vi "ldr motor sir.vi"() -> ()   [LabVIEW 2020]
uses:
  <vilib>/MakerHub/LINX/Private/Device/Type Defs/Stimulus Pulse.ctl
  <vilib>/MakerHub/LINX/Public/Peripherals/Analog/Analog Read 1 Chan.vi
  <vilib>/MakerHub/LINX/Public/Peripherals/Digital/Digital Write 1 Chan.vi
  <vilib>/MakerHub/LINX/Public/Peripherals/PWM/PWM Set Duty Cycle 1 Chan.vi
  <vilib>/MakerHub/LINX/Public/Peripherals/Analog/Analog Read N Chans.vi
  <vilib>/MakerHub/LINX/Public/Peripherals/Digital/Digital Write N Chans.vi
  <vilib>/MakerHub/LINX/Private/Local IO/LinxAnalogRead.vi
  <vilib>/MakerHub/LINX/Public/Utilities/Check Channel.vi
  <vilib>/MakerHub/LINX/Private/Local IO/LinxDigitalWrite.vi
  <vilib>/MakerHub/LINX/Public/Utilities/Open Serial.vi
  <vilib>/MakerHub/LINX/Private/Utilties/Generate Error.vi
  <vilib>/MakerHub/LINX/Public/Peripherals/PWM/PWM Set Duty Cycle N Chans.vi
  <vilib>/MakerHub/LINX/Private/Device/Device.lvlib
  <vilib>/MakerHub/LINX/LMH-LINX.lvlib
panel:
  in  "Serial Port":refnum<visa-resource-name>="N/A"
  in  "stop of ldr while":bool
  out "Light Intensity":dbl
  out "voltage across ldr":dbl
  in  "Knob":dbl(knob) scale=0.0..1.0
  out "Pulse Width (uS)":u32
  out "U1 Distance(cm)":u32
  out "Waveform Chart u1":dbl(graph)
  in  "Trigger":u8
  in  "Echo":u8
  in  "LDR Analog pin":u8
  in  "IN2 Motor":u8
  in  "Enable PWM Channel for  motor":u8
  in  "Trigger 2":u8
  in  "Echo 2":u8
  out "Pulse Width (uS) 2":u32
  out "U1 Distance(cm) 2":u32
  out "Waveform Chart u1\n 2":dbl(graph)
  in  "IN1 Motor":u8
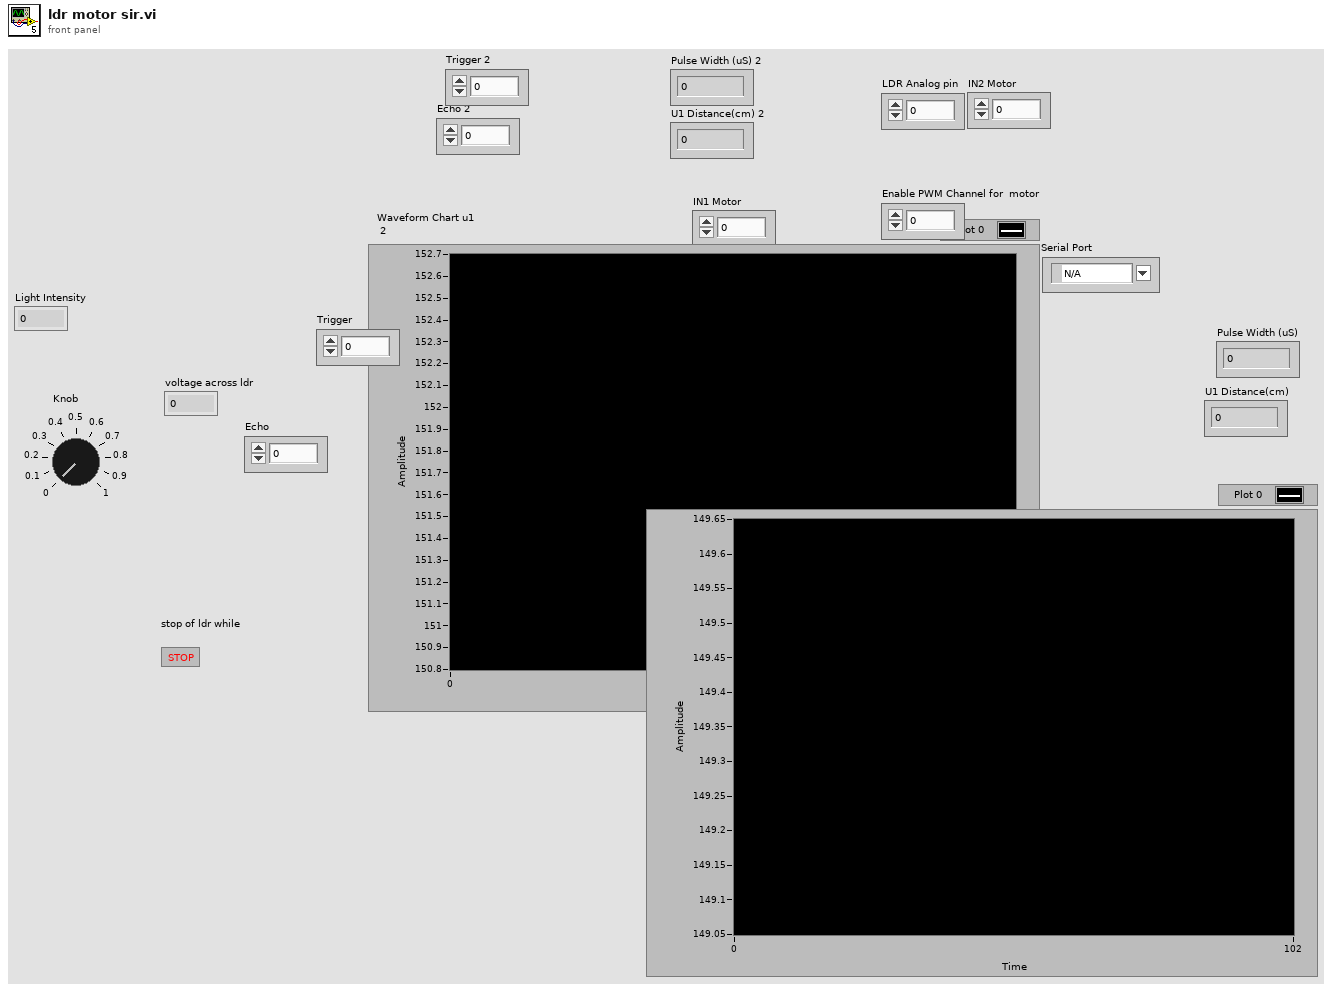
[diagram p1: front panel]
types:
  T1 = typedef "LMH-LINX.lvlib/LINX Ref.ctl" = cluster{"IO":T2, "Interface":T3, "LINX Device Config":T4}
  T2 = typedef "LMH-LINX.lvlib/Platform.ctl" = enum16{"Remote", "Local"}
  T3 = typedef "LMH-LINX.lvlib/Interface.ctl" = enum16{"Serial", "TCP"}
  T4 = typedef "LMH-LINX.lvlib/Device.lvlib/LINX Device Config.ctl" = cluster{"Interface":T3, "COM Port":refnum<visa-resource-name>, "TCP Configuration":T5, "Device Family":u8, "Device ID":u8, "Device Name":string, "TCP Ref":refnum<k5>, "Channels":T6}
  T5 = typedef "LMH-LINX.lvlib/Device.lvlib/TCP Config.ctl" = cluster{"IP Address":string, "Port":u16}
  T6 = typedef "LMH-LINX.lvlib/Channels.ctl" = cluster{"DI":u8[], "DO":u8[], "AI":u8[], "AO":u8[], "PWM":u8[], "QE":u8[], "UART":u8[], "I2C 2":u8[], "SPI":u8[], "CAN":u8[], "Servo":u8[], "AI Ref (V)":dbl, "AI Resolution (Bits)":u8, "AO Ref (V)":dbl, "AO Resolution (Bits)":u8}
  T7 = typedef "LMH-LINX.lvlib/Device.lvlib/Stimulus Pulse.ctl" = enum16{"None", "Active Low", "Active High"}
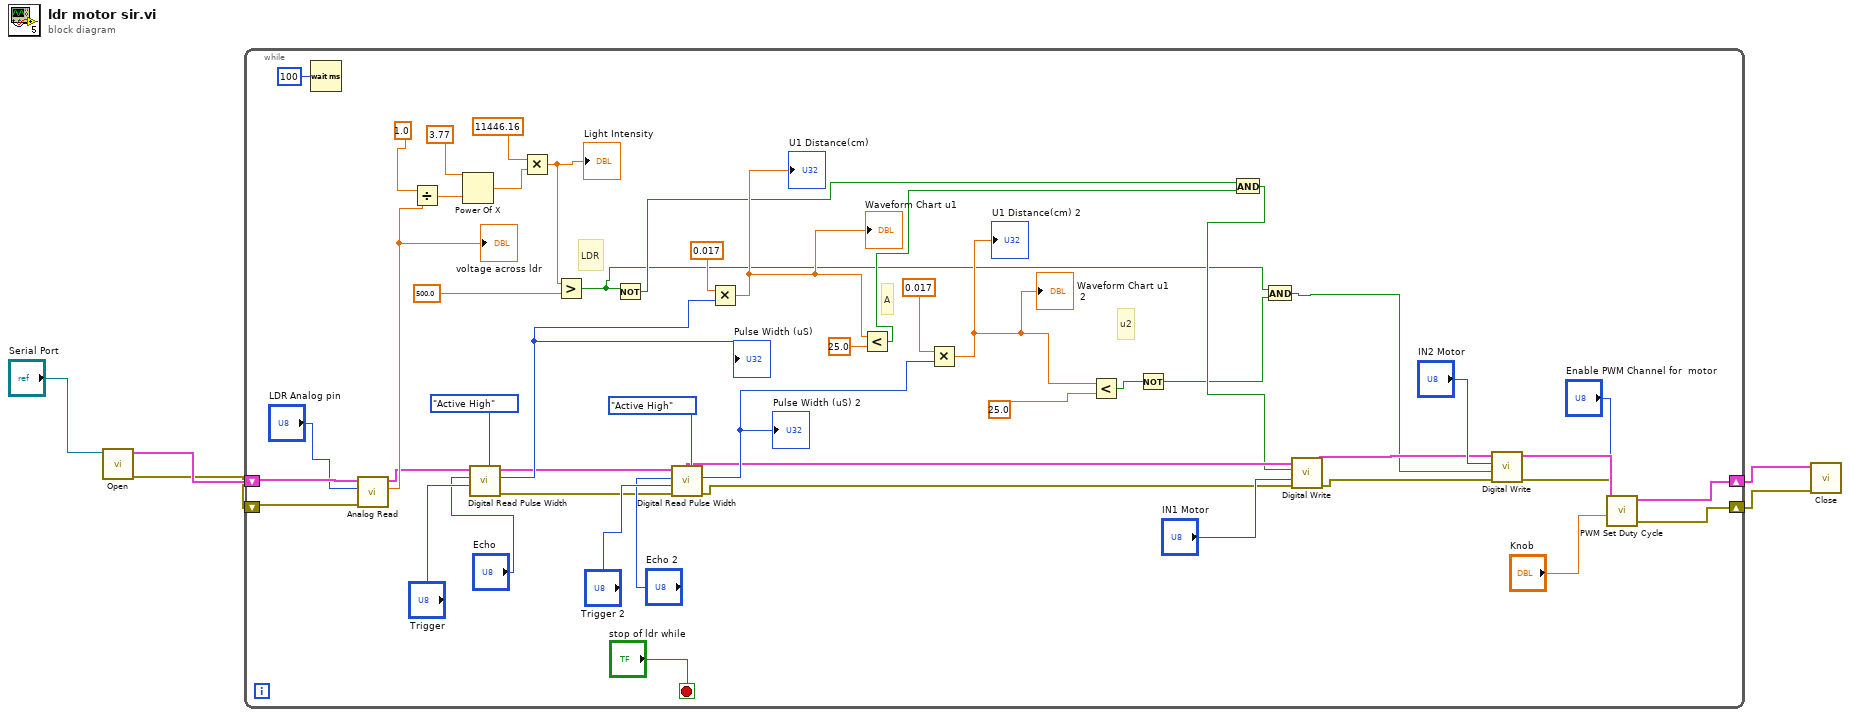
[diagram p0: block diagram]
diagram:
  n1 = call-poly <vilib>:"Open.vi"("Serial Port"="Serial Port") -> ("Error Out"=w2:errorcluster, "LINX Resource"=w3:T1)  [unwired: 8 in, 1 out]
  n2 = while {
    shift-right: [w34] -> w5
    shift-left: w3 -> [w54]
    shift-right: [w33] -> w4
    shift-left: w2 -> [w53]
    stop <- "stop of ldr while" stop-if-true
    # "u2"
    # "A"
    # "LDR"
    n3 = Wait (ms)(milliseconds to wait=u32 100) -> ()  [unwired: 1 out]
    n4 = call-poly <vilib>:"Analog Read.vi"("Error In"=w53, "Analog Channel"="LDR Analog pin", "LINX Resource"=w54) -> ("Voltage"=w45:dbl, "LINX Resource"=w32:T1)  [unwired: 5 in, 2 out]
    "voltage across ldr" <- w45
    n5 = Divide(x=1.0, y=w45) -> (x/y=w49:dbl)
    n6 = Power Of X(1:w49, 2:3.77 ("y")) -> (0:w47:dbl)
    n7 = call <vilib>:"Digital Read Pulse Width.vi"("Stimulus Pulse (Active High)"=Stimulus_Pulse."Active High", "DO Channel"="Trigger", "DI Channel"="Echo", "LINX Resource"=w32) -> ("Error Out"=w17:errorcluster, "Pulse Width (uS)"=w39:u32, "LINX Resource"=w18:T1)  [unwired: 5 in]
    "Pulse Width (uS)" <- w39
    n8 = Multiply(x=11446.16, y=w47) -> (x*y=w31:dbl)
    "Light Intensity" <- w31
    n9 = Greater?(x=w31, y=500.0) -> (0:w7:bool)
    n10 = Not(x=w7) -> (.not. x?=w12:bool)
    n11 = call <vilib>:"Digital Read Pulse Width.vi"("Stimulus Pulse (Active High)"=Stimulus_Pulse."Active High", "Error In"=w17, "DO Channel"="Trigger 2", "DI Channel"="Echo 2", "LINX Resource"=w18) -> ("Error Out"=w15:errorcluster, "Pulse Width (uS)"=w20:u32, "LINX Resource"=w16:T1)  [unwired: 4 in]
    "Pulse Width (uS) 2" <- w20
    n12 = Multiply(x=0.017, y=w39) -> (x*y=w38:dbl)
    "U1 Distance(cm)" <- w38
    "Waveform Chart u1" <- w38
    n13 = Less?(x=w38, y=25.0) -> (x < y?=w11:bool)
    n14 = Multiply(x=0.017, y=w20) -> (x*y=w22:dbl)
    "U1 Distance(cm) 2" <- w22
    "Waveform Chart u1\n 2" <- w22
    n15 = Less?(x=w22, y=25.0) -> (x < y?=w8:bool)
    n16 = Not(x=w8) -> (.not. x?=w6:bool)
    n17 = And(x=w12, y=w11) -> (x .and. y?=w10:bool)
    n18 = And(x=w7, y=w6) -> (x .and. y?=w9:bool)
    n19 = call-poly <vilib>:"Digital Write.vi"("Error In"=w15, "Output Value"=w10, "DO Channel"="IN1 Motor", "LINX Resource"=w16) -> ("Error Out"=w13:errorcluster, "LINX Resource"=w14:T1)  [unwired: 6 in]
    n20 = call-poly <vilib>:"Digital Write.vi"("Error In"=w13, "Output Value"=w9, "DO Channel"="IN2 Motor", "LINX Resource"=w14) -> ("Error Out"=w43:errorcluster, "LINX Resource"=w44:T1)  [unwired: 6 in]
    n21 = call-poly <vilib>:"PWM Set Duty Cycle.vi"("Error In"=w43, "Duty Cycle (0-1)"="Knob", "PWM Channel"="Enable PWM Channel for  motor", "LINX Resource"=w44) -> ("Error Out"=w33:errorcluster, "LINX Resource"=w34:T1)  [unwired: 6 in]
  }
  n22 = call <vilib>:"Close.vi"("Error In"=w4, "LINX Resource"=w5) -> ()  [unwired: 9 in, 1 out]
